vi "Get PPL with version.vi"(11 "Plugin path":path=path "Plugin path") -> (2 "Plugin":string[](array[string]), 3 "Version":string[](array[string]))   [LabVIEW 2025, in "HW Engine.lvlib" / "HW Engine.lvclass"]
uses:
  HW Engine.lvclass
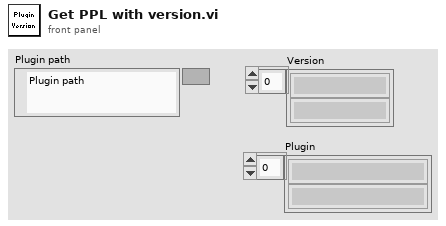
[diagram p1: front panel]
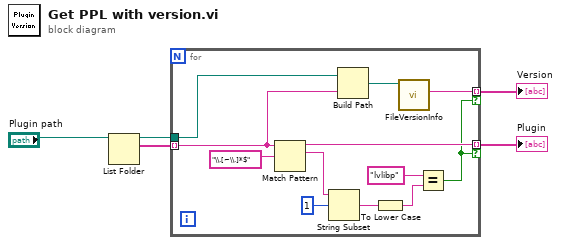
[diagram p0: block diagram]
diagram:
  n1 = List Folder(path="Plugin path") -> (path out=w2:path, filenames=w5:string[])  [unwired: 3 in, 2 out]
  n2 = for {
    tunnel: w5 -> [w7] mode=indexing
    tunnel: [w11] -> w4 mode=indexing if=w9
    tunnel: [w10] -> w1 mode=indexing if=w9
    tunnel: w2 -> [w8]
    n3 = Match Pattern(string=w7, regular expression="\\.[~\\.]*$") -> (before substring=w11:string, match substring=w16:string)  [unwired: 3 out]
    n4 = String Subset(string=w16, offset (0)=1) -> (substring=w14:string)  [unwired: 1 out]
    n5 = Build Path(base path=w8, name or relative path=w7) -> (appended path=w6:path)
    n6 = To Lower Case(string=w14) -> (all lower case string=w13:string)
    n7 = call <vilib>:"FileVersionInfo.vi"("Application Path in"=w6) -> ("File Version Info"=w10:string)  [unwired: 7 in, 3 out]
    n8 = Equal?(x="lvlibp", y=w13) -> (x = y?=w9:bool)
  }
  "Plugin" <- w4
  "Version" <- w1
